vi "Get Toggle Bit.vi"(8 "error in":errorcluster, 11 "CANopen Response Message in":refnum<class "CANopen Response Message.lvclass">) -> (0 "error out":errorcluster, 2 "Toggle-Bit":bool, 3 "CANopen Response Message out":refnum<class "CANopen Response Message.lvclass">)   [LabVIEW 2024, in "CANopen Master.lvlib" / "CANopen Response Message.lvclass"]
uses:
  CANopen Response Message.lvclass
  CANopen Response Message.lvclass/CANopen Response Message.ctl
  CANopen Message/CANopen Message.lvclass
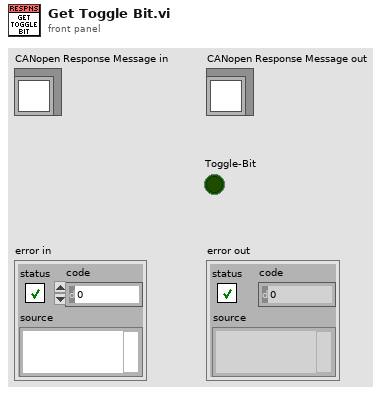
[diagram p1: front panel]
types:
  T1 = typedef "CANopen Master.lvlib/CANopen Response Message.lvclass/Server Command Specifier.ctl" = enum8{"Upload Segment Response", "Download Segment Response", "Initiate Upload Response", "Initiate Download Response", "Heartbeat", "Block Download"}
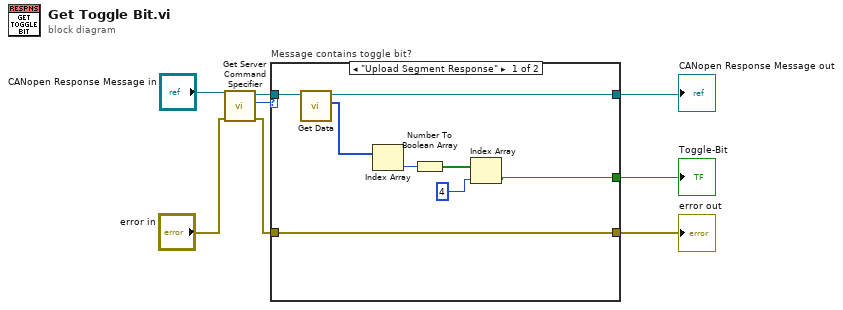
[diagram p0: block diagram]
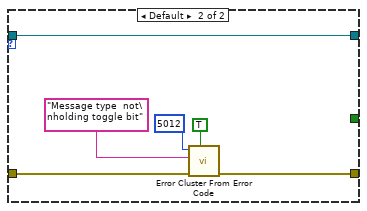
[diagram p2: hidden frame]
diagram:
  n1 = call-dynamic "Get Server Command Specifier.vi"("error in"="error in", "CANopen Response in"="CANopen Response Message in") -> ("error out"=w2:errorcluster, "Server Command Specifier"=w7:T1, "CANopen Response out"=w5:refnum<class "CANopen Response Message.lvclass">)  [unwired: 7 in]
  n2 = case "Message contains toggle bit?" shown="\"Upload Segment Response\"" w7 {
    tunnel: w2 -> [w16 w22]
    tunnel: [w16 w21] -> w6
    tunnel: w5 -> [w15 w17]
    tunnel: [w9 w17] -> w4
    tunnel: [w10 _] -> w1
    frame "Upload Segment Response" {
      n3 = call "Get Data.vi"("CANopen Message in"=w15) -> ("Data"=w14:u8[], "CANopen Message out"=w9:refnum<class "CANopen Response Message.lvclass">)  [unwired: 9 in]
      n4 = Index Array(array=w14) -> (element=w13:u8)  [unwired: 1 in]
      n5 = Number To Boolean Array(number=w13) -> (Boolean array=w12:bool[])
      n6 = Index Array(array=w12, index=4) -> (element=w10:bool)
    }
    frame Default {
      n7 = call <vilib>:"Error Cluster From Error Code.vi"("show call chain? (False)"=TRUE, "error in (no error)"=w22, "error message (\"\")"="Message type  not\nholding toggle bit" ("error message (\"\")"), "error code (0)"=5012) -> ("error out"=w21:errorcluster)  [unwired: 5 in]
    }
  }
  "error out" <- w6
  "CANopen Response Message out" <- w4
  "Toggle-Bit" <- w1
